vi "CTR-Initialize.vi"(0 "Config":T1={"enabled"=FALSE, "Hi ticks"=5, "Low ticks"=4995, "Idle state"=10214, "Delay ticks"=0} {"Idle state" items=["High"=10192, "Low"=10214]; "Low ticks" max=1}, 7 "task":refnum<k21>, 11 "error in (no error)":errorcluster) -> (8 "Counter Task":T2={"task"="Counter"}, 15 "error out":errorcluster)   [LabVIEW 2020]
uses:
  Typedefs/CTR-Task Specification.ctl
  Typedefs/CTR-Config.ctl
  <vilib>/DAQmx/create/channels.llb/DAQmx Create Channel (CO-Pulse Generation-Ticks).vi
  <vilib>/DAQmx/configure/timing.llb/DAQmx Timing (Implicit).vi
  <vilib>/DAQmx/configure/trigger.llb/DAQmx Start Trigger (Digital Edge).vi
  <resource>/objmgr/daqmx.rc
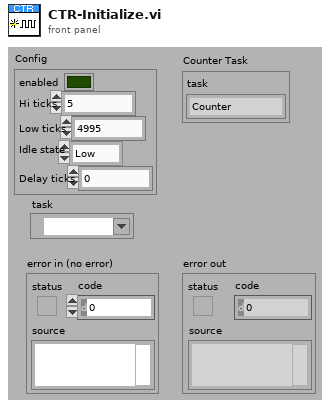
[diagram p1: front panel]
types:
  T1 = typedef "CTR-Config.ctl" = cluster{"enabled":bool, "Hi ticks":u32, "Low ticks":u32, "Idle state":i32, "Delay ticks":u32}
  T2 = typedef "CTR-Task Specification.ctl" = cluster{"task":string}
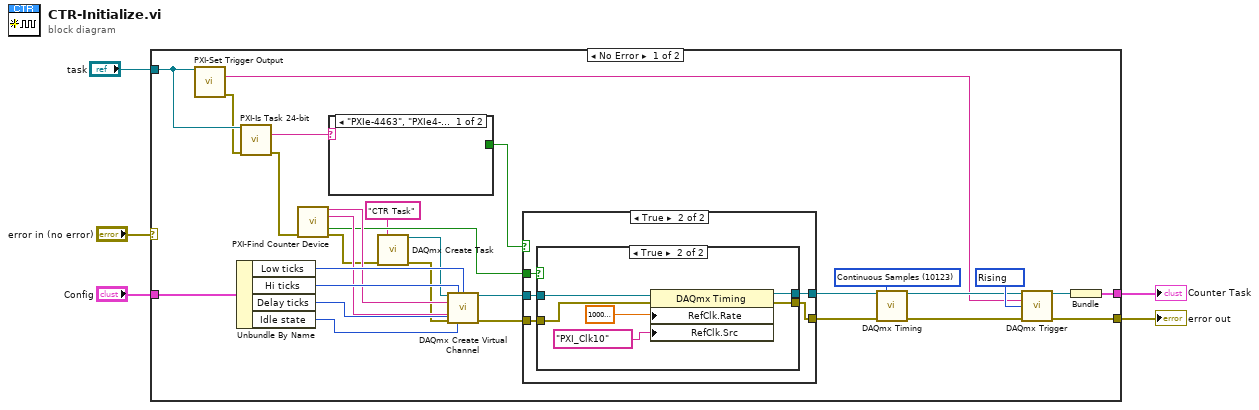
[diagram p0: block diagram]
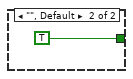
[diagram p2: hidden frame]
diagram:
  n1 = case shown="No Error" "error in (no error)" {
    selector: "error in (no error)" -> [_ w51]
    tunnel: [w34 w51] -> w5
    tunnel: [w15 _] -> w3
    tunnel: "Config" -> [w14 _]
    tunnel: "task" -> [w13 _]
    frame No Error {
      w32 = 10280 items=["Rising"=10280, "Falling"=10171] ("Trigger Edge")
      w33 = 10123 items=["Finite Samples"=10178, "Continuous Samples"=10123] ("sample mode")
      n2 = call "PXI-Set Trigger Output.vi"("Task in"=w13) -> ("Trigger Terminal"=w12:string, "error out"=w11:errorcluster)  [unwired: 12 in, 1 out]
      n3 = Unbundle By Name(w14) -> ("Low ticks"=w25:u32, "Hi ticks"=w24:u32, "Delay ticks"=w23:u32, "Idle state"=w22:i32)
      n4 = call "PXI-Is Task 24-bit.vi"("task"=w13, "error in (no error)"=w11) -> ("Product Type"=w19:string, "error out"=w10:errorcluster)  [unwired: 8 in, 4 out]
      n5 = call "PXI-Find Counter Device.vi"("error in (no error)"=w10) -> ("Counter Channel"=w21:tag, "RefClk.Src"=w20:tag, "Is M-series board"=w17:bool, "error out"=w7:errorcluster)  [unwired: 10 in, 1 out]
      n6 = case shown="\"PXIe-4463\", \"PXIe4-4464\"" w19 {
        tunnel: [_ TRUE] -> w18
        frame "PXIe-4463", "PXIe4-4464" {
        }
        frame "", Default {
        }
      }
      n7 = call <vilib>:"DAQmx Create Task.vi"("new task name"="CTR Task" ("name to assign"), "error in"=w7) -> ("task out"=w8:refnum<k21>, "error out"=w6:errorcluster)  [unwired: 12 in]
      n8 = call-poly <vilib>:"DAQmx Create Virtual Channel.vi"("task in"=w8, "high ticks"=w24, "low ticks"=w25, "counter"=w21, "source of ticks"=w20, "error in"=w6, "idle state"=w22, "initial delay"=w23) -> ("task out"=w26:refnum<k21>, "error out"=w27:errorcluster)  [unwired: 6 in]
      n9 = case shown="True" w18 {
        tunnel: [w37 w42] -> w31
        tunnel: [w36 w41] -> w30
        tunnel: w27 -> [w36 w40]
        tunnel: w26 -> [w37 w39]
        tunnel: w17 -> [_ w38]
        frame False {
        }
        frame True {
          n10 = case shown="True" w38 {
            tunnel: [w44 w50] -> w42
            tunnel: [w43 w49] -> w41
            tunnel: w40 -> [w43 w48]
            tunnel: w39 -> [w44 w47]
            frame False {
            }
            frame True {
              n11 = property class="DAQmx Timing"(reference=w47, error in=w48, "RefClk.Rate"=10000000.0, "RefClk.Src"=tag "PXI_Clk10") -> (reference out=w50:refnum<k21>, error out=w49:errorcluster)
            }
          }
        }
      }
      n12 = call-poly <vilib>:"DAQmx Timing.vi"("task/channels in"=w31, "sample mode"=w33, "error in"=w30) -> ("task out"=w29:refnum<k21>, "error out"=w28:errorcluster)  [unwired: 11 in]
      n13 = call-poly <vilib>:"DAQmx Trigger.vi"("task/channels in"=w29, "source"=w12, "edge"=w32, "error in"=w28) -> ("task out"=w16:refnum<k21>, "error out"=w34:errorcluster)  [unwired: 10 in]
      n14 = Bundle("task out"=w16) -> (w15:cluster{"task out":refnum<k21>})  [unwired: 1 in]
    }
    frame Error {
    }
  }
  "error out" <- w5
  "Counter Task" <- w3
